vi "Create Message Setter (from Accessor).vi"(8 "error in (no error)":errorcluster, 10 "RPC Message Name":string, 11 "RPC Messages Folder (ProjectItem) in":refnum<vi>) -> (0 "error out":errorcluster, 1 "Created ?":bool, 2 "Getter VI out":refnum<vi>, 3 "RPC Messages Folder (ProjectItem) out":refnum<vi>)   [LabVIEW 2019, in "gRPC Scripting Tools.lvlib"]
uses:
  gRPC Scripting Tools.lvlib
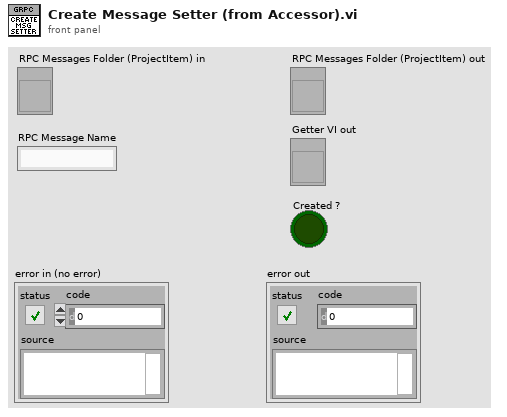
[diagram p1: front panel]
types:
  T1 = enum32{"invalid VI type", "Standard VI", "Control VI", "Global VI", "Polymorphic VI", "Configuration VI", "SubSystem", "Facade VI", "Method VI"}
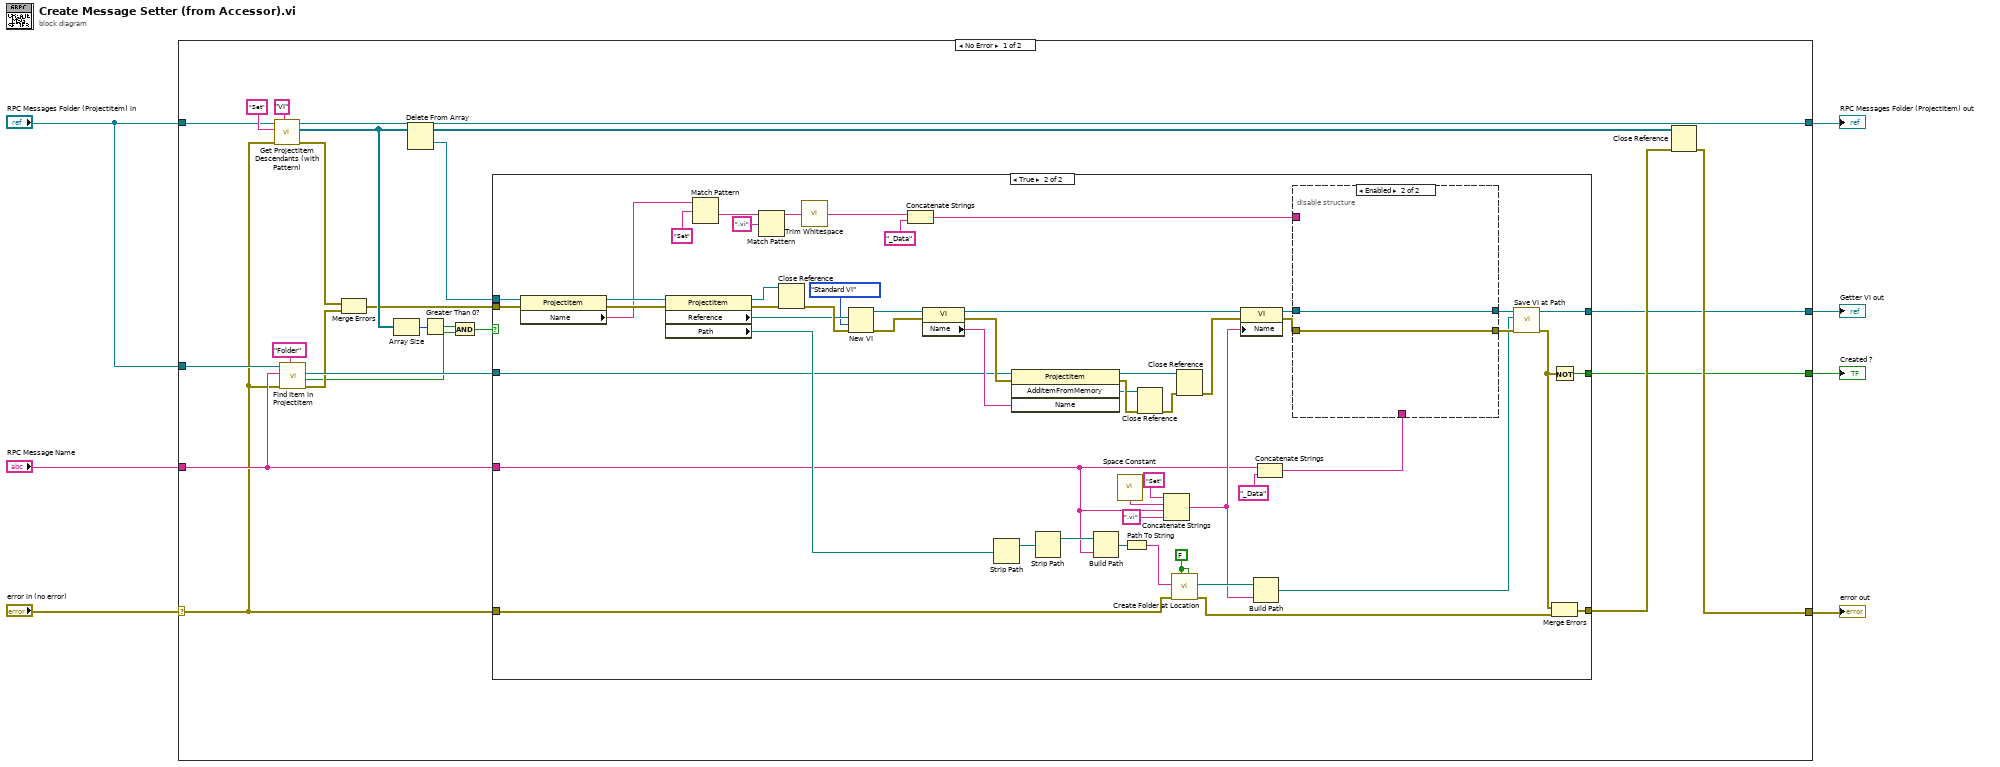
[diagram p0: block diagram]
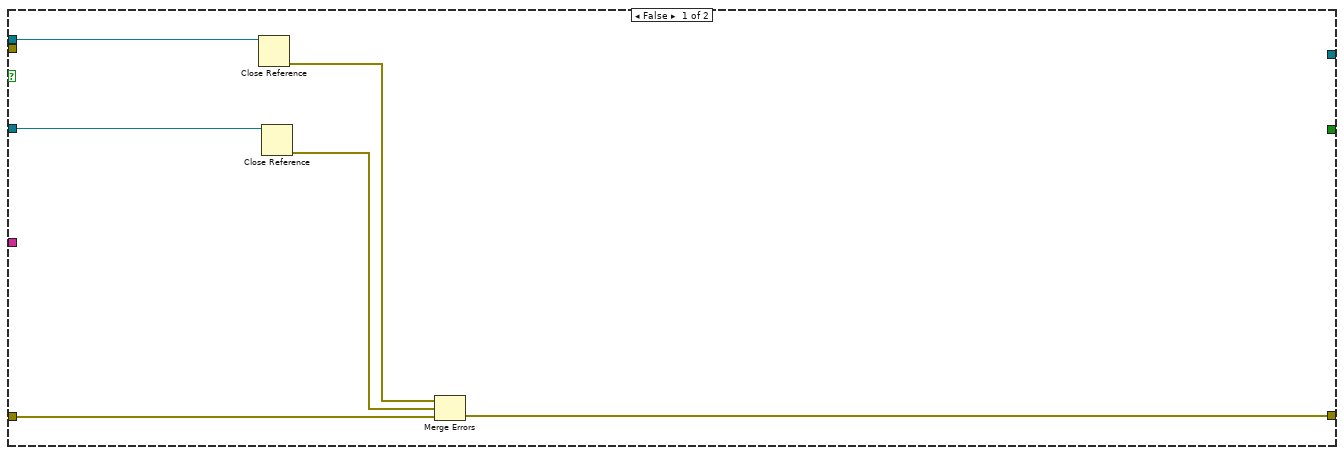
[diagram p2: hidden frame]
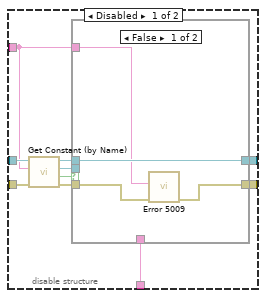
[diagram p3: hidden frame]
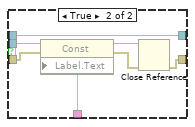
[diagram p4: hidden frame]
diagram:
  n1 = case shown="No Error" "error in (no error)" {
    selector: "error in (no error)" -> [w13 w114]
    tunnel: "RPC Message Name" -> [w25 _]
    tunnel: "RPC Messages Folder (ProjectItem) in" -> [w23 _]
    tunnel: "RPC Messages Folder (ProjectItem) in" -> [w18 w113]
    tunnel: [w11 w114] -> w4
    tunnel: [w10 w113] -> w3
    tunnel: [w9 _] -> w2
    tunnel: [w8 _] -> w1
    frame No Error {
      n2 = call "Get ProjectItem Descendants (with Pattern).vi"("Type"="VI", "error in (no error)"=w13, "Pattern"="Set", "ProjectItem in"=w18) -> ("error out"=w17:errorcluster, "ProjectItem descendents"=w24:refnum<vi>[], "ProjectItem out"=w10:refnum<vi>)  [unwired: 5 in]
      n3 = call "Find Item in ProjectItem.vi"("Item Type"="Folder", "error in (no error)"=w13, "Name"=w25, "ProjectItem in"=w23) -> ("error out"=w16:errorcluster, "Found ?"=w15:bool, "Item Refnum out"=w21:refnum<vi>)  [unwired: 4 in, 1 out]
      n4 = Merge Errors(w17, w16) -> (w14:errorcluster)
      n5 = Array Size(array=w24) -> (size(s)=w22:i32)
      n6 = Delete From Array(array=w24) -> (deleted portion=w27:refnum<vi>, array with subset deleted=w30:refnum<vi>[])  [unwired: 2 in]
      n7 = Greater Than 0?(x=w22) -> (x > 0?=w20:bool)
      n8 = And(x=w20, y=w15) -> (x .and. y?=w19:bool)
      n9 = case shown="True" w19 {
        tunnel: w25 -> [_ w45]
        tunnel: [w33 w86] -> w12
        tunnel: [_ w42] -> w8
        tunnel: w27 -> [w36 w58]
        tunnel: [_ w68] -> w9
        tunnel: w21 -> [w31 w63]
        tunnel: w13 -> [w32 w62]
        tunnel: w14 -> [_ w57]
        frame False {
          n10 = Close Reference(reference=w36) -> (error out=w34:errorcluster)  [unwired: 1 in]
          n11 = Close Reference(reference=w31) -> (error out=w35:errorcluster)  [unwired: 1 in]
          n12 = Merge Errors(w34, w35, w32) -> (w33:errorcluster)
        }
        frame True {
          w84 = FALSE ("Use Relative (F)")
          n13 = property class="ProjectItem"(reference=w58, error in=w57) -> (reference out=w56:refnum<vi>, error out=w55:errorcluster, "Name"=w54:string)
          n14 = property class="ProjectItem"(reference=w56, error in=w55) -> (reference out=w89:refnum<vi>, error out=w87:errorcluster, "Reference"=w74:refnum<vi>, "Path"=w80:path)
          n15 = Match Pattern(string=w54, regular expression="Set") -> (after substring=w52:string)  [unwired: 1 in, 3 out]
          n16 = Match Pattern(string=w52, regular expression=".vi") -> (before substring=w39:string)  [unwired: 1 in, 3 out]
          n17 = Close Reference(reference=w89, error in (no error)=w87) -> (error out=w88:errorcluster)
          n18 = call <vilib>:"Trim Whitespace.vi"("string"=w39) -> ("trimmed string"=w50:string)  [unwired: 1 in]
          n19 = New VI(8:w88, 9:T1."Standard VI" ("vi type (standard vi)"), 10:w74) -> (0:w73:errorcluster, 3:w71:refnum<vi>)  [unwired: 1 in, 3 out]
          n20 = Concatenate Strings(w50, "_Data" ("string")) -> (w37:string)
          n21 = property class="VI"(reference=w71, error in=w73) -> (reference out=w81:refnum<vi>, error out=w82:errorcluster, "Name"=w75:string)
          n22 = Strip Path(path=w80) -> (stripped path=w76:path)  [unwired: 1 out]
          n23 = invoke class="ProjectItem" method="AddItemFromMemory"(reference=w63, error in=w82, "Name"=w75) -> (reference out=w70:refnum<vi>, error out=w61:errorcluster, "AddItemFromMemory"=w60:refnum<vi>)  [unwired: 1 in, 1 out]
          n24 = Strip Path(path=w76) -> (stripped path=w77:path)  [unwired: 1 out]
          n25 = Build Path(base path=w77, name or relative path=w45) -> (appended path=w78:path)
          n26 = call <vilib>:"Space Constant.vi"() -> ("String"=w66:string)
          n27 = Path To String(path=w78) -> (string=w79:string)
          n28 = Close Reference(reference=w60, error in (no error)=w61) -> (error out=w59:errorcluster)
          n29 = Concatenate Strings("Set" ("string"), w66, w45, ".vi" ("string")) -> (w64:string)
          n30 = call "Create Folder at Location.vi"("Override existing (F)"=w84, "Use Relative (F)"=w84, "Error In"=w62, "Path"=w79) -> ("Error Out"=w85:errorcluster, "Full path out"=w83:path)  [unwired: 5 in, 1 out]
          n31 = Close Reference(reference=w70, error in (no error)=w59) -> (error out=w69:errorcluster)
          n32 = property class="VI"(reference=w81, error in=w69, "Name"=w64) -> (reference out=w48:refnum<vi>, error out=w47:errorcluster)
          n33 = Build Path(base path=w83, name or relative path=w64) -> (appended path=w41:path)
          n34 = Concatenate Strings(w45, "_Data" ("string")) -> (w44:string)
          n35 = disable-structure shown="Enabled" {
            disable-tunnel: w48 -> [w98 w112]
            disable-tunnel: w47 -> [w97 w111]
            disable-tunnel: w44 -> [w96 _]
            disable-tunnel: [w94 w111] -> w43
            disable-tunnel: [w91 w112] -> w38
            disable-tunnel: w37 -> [w90 _]
            frame Disabled {
              n36 = call "Get Constant (by Name).vi"("error in (no error)"=w97, "Constant Label"=w90, "Owner VI in"=w98) -> ("error out"=w95:errorcluster, "Found ?"=w93:bool, "Const ref out"=w99:refnum<vi>, "Owner VI out"=w92:refnum<vi>)  [unwired: 5 in]
              n37 = case shown="False" w93 {
                tunnel: w99 -> [_ w110]
                tunnel: w96 -> [_ w109]
                tunnel: w95 -> [w102 w108]
                tunnel: [w101 w105] -> w94
                tunnel: w92 -> [w103 w104]
                tunnel: [w103 w104] -> w91
                tunnel: w90 -> [w100 _]
                frame False {
                  n38 = call "Error 5009.vi"("error in (no error)"=w102, "Cluster Definition Constant"=w100) -> ("error out"=w101:errorcluster)  [unwired: 9 in]
                }
                frame True {
                  n39 = property class="Const"(reference=w110, error in=w108, "Label.Text"=w109) -> (reference out=w107:refnum<vi>, error out=w106:errorcluster)
                  n40 = Close Reference(reference=w107, error in (no error)=w106) -> (error out=w105:errorcluster)
                }
              }
            }
            frame Enabled {
            }
          }
          n41 = call "Save VI at Path.vi"("error in (no error)"=w43, "Path"=w41, "VI in"=w38) -> ("error out"=w40:errorcluster, "VI out"=w42:refnum<vi>)  [unwired: 6 in, 1 out]
          n42 = Not(x=w40) -> (.not. x?=w68:bool)
          n43 = Merge Errors(w40, w85) -> (w86:errorcluster)
        }
      }
      n44 = Close Reference(reference=w30, error in (no error)=w12) -> (error out=w11:errorcluster)
    }
    frame Error {
    }
  }
  "error out" <- w4
  "RPC Messages Folder (ProjectItem) out" <- w3
  "Created ?" <- w2
  "Getter VI out" <- w1
